vi "PTC04_SN_Array.vi"(8 "error in (no error)":errorcluster, 11 "IN":T1={"step name 1"="", "updata 2"="1000", "limitdata 3"="", "load vi name 4"="", "parameter 5"=""}) -> (0 "error out":errorcluster, 2 "Register?":bool, 3 "Cluster":T2)   [LabVIEW 2013]
uses:
  Global constant.vi
panel:
  out "type string":i16[](array[numeric])
  out "data string":string
  out "GetMainHardwareID":variant
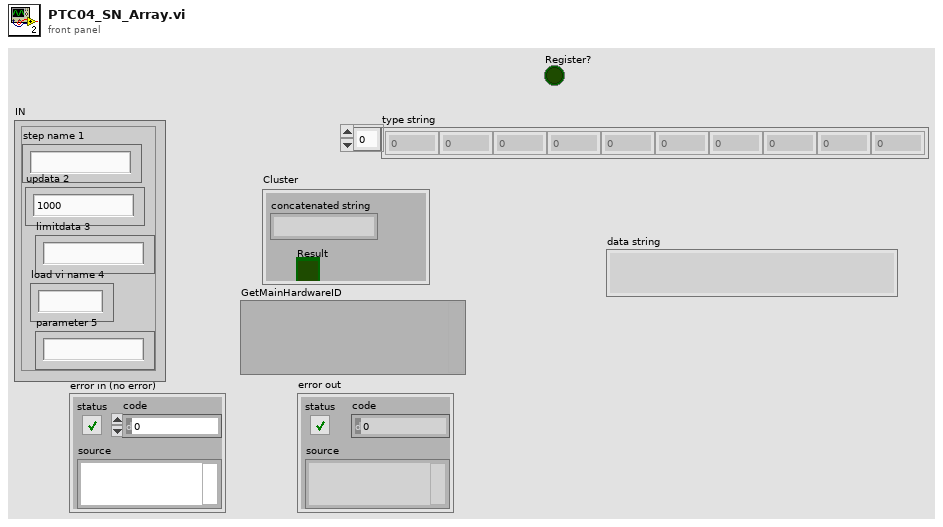
[diagram p1: front panel]
types:
  T1 = cluster{"step name 1":string, "updata 2":string, "limitdata 3":string, "load vi name 4":string, "parameter 5":string}
  T2 = cluster{"concatenated string":string, "Result":bool}
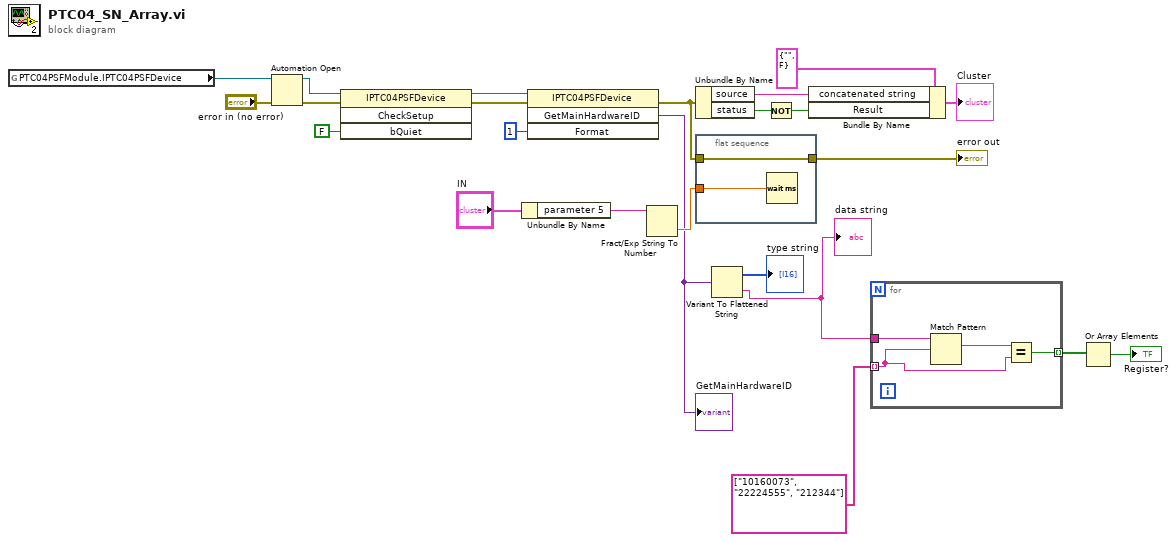
[diagram p0: block diagram]
diagram:
  n1 = global read "Global constant.vi" "PTC04PSFModule.IPTC04PSFDevice"() -> (w19:refnum<k7>)
  n2 = Automation Open(error in (no error)="error in (no error)", Automation Refnum=w19) -> (Automation Refnum=w17:refnum<k7>, error out=w16:errorcluster)  [unwired: 2 in]
  n3 = invoke class="IPTC04PSFDevice" method="CheckSetup"(reference=w17, error in=w16, "bQuiet"=FALSE) -> (reference out=w10:refnum<k7>, error out=w9:errorcluster)  [unwired: 1 in, 2 out]
  n4 = Unbundle By Name("IN") -> ("parameter 5"=w20:string)
  n5 = invoke class="IPTC04PSFDevice" method="GetMainHardwareID"(reference=w10, error in=w9, "Format"=1) -> (error out=w7:errorcluster, "GetMainHardwareID"=w6:variant)  [unwired: 1 in, 2 out]
  "GetMainHardwareID" <- w6
  n6 = Fract/Exp String To Number(string=w20) -> (number=w21:dbl)  [unwired: 3 in, 1 out]
  n7 = Unbundle By Name(w7) -> ("source"=w12:string, "status"=w14:bool)
  n8 = flat-sequence {
    tunnel: w21 -> [w26]
    tunnel: w7 -> [w25]
    tunnel: [w25] -> w11
    frame #0 {
      n9 = Wait (ms)(milliseconds to wait=w26) -> ()  [unwired: 1 out]
    }
  }
  n10 = Variant To Flattened String(Variant=w6) -> (data string=w4:string, 1:→"type string":i16[])
  "data string" <- w4
  n11 = Not(x=w14) -> (.not. x?=w13:bool)
  n12 = Bundle By Name(cluster=T2 {"concatenated string"="", "Result"=FALSE} ("Cluster"), "concatenated string"=w12, "Result"=w13) -> (→"Cluster":T2)
  n13 = for {
    tunnel: w4 -> [w30]
    tunnel: string[] ["10160073", "22224555", "212344"] -> [w28] mode=indexing
    tunnel: [w27] -> w2 mode=indexing
    n14 = Match Pattern(string=w30, regular expression=w28) -> (match substring=w29:string)  [unwired: 1 in, 3 out]
    n15 = Equal?(x=w29, y=w28) -> (x = y?=w27:bool)
  }
  n16 = Or Array Elements(Boolean array=w2) -> (logical OR=→"Register?":bool)
  "error out" <- w11
